vi "Initialize Shared Memory.vi"   [LabVIEW 2013]
doc: "This template VI demonstrates a default initialization that creates and configures a shared memory file in Linux RT. In an unmodified install of Linux RT, the shared memory files will be located at /dev/shm using the name provided to the Initialize Shared Memory VI.\n\nThe template sets the size of the shared memory file to be the size of one page in memory. This avoids page framentation, which may improve performance by reducing the number of interactions with the OS's paging table. However, the size can be set to any value >= 0 if large data sets are required."
uses:
  Classes/Shared Memory/Public/Controls/file mode.ctl
  Classes/Shared Memory/Shared Memory.lvclass
types:
  T1 = typedef "Linux RT IPC.lvlib/Shared Memory.lvlib/Shared Memory.lvclass/file mode.ctl" = enum16{"open", "create/replace"}
  T2 = typedef "Linux RT IPC.lvlib/Shared Memory.lvlib/Shared Memory.lvclass/reference.ctl" = refnum<data-value>
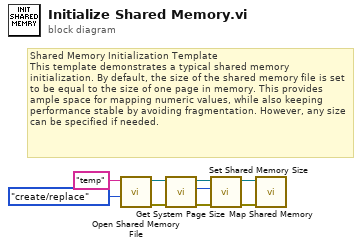
[diagram p0: block diagram]
diagram:
  # "Shared Memory Initialization Template\nThis template demonstrates a typical shared memory initialization. By default, the size of the shared memory file is set to be equal to the size of one page in memory. This provides ample space for mapping numeric values, while also keeping performance stable by avoiding fragmentation. However, any size can be specified if needed."
  n1 = call "Open Shared Memory File.vi"("file mode (open)"=file_mode."create/replace" ("file mode (default: open)"), "shared memory name"="temp") -> ("error out"=w6:errorcluster, "shared memory out"=w7:T2)  [unwired: 8 in]
  n2 = call "Get System Page Size.vi"("error in (no error)"=w6, "shared memory in"=w7) -> ("error out"=w1:errorcluster, "page size (bytes)"=w2:u32, "shared memory out"=w5:T2)  [unwired: 7 in]
  n3 = call "Set Shared Memory Size.vi"("error in (no error)"=w1, "size (bytes)"=w2, "shared memory in"=w5) -> ("error out"=w3:errorcluster, "shared memory out"=w4:T2)  [unwired: 7 in]
  n4 = call "Map Shared Memory.vi"("error in (no error)"=w3, "shared memory in"=w4) -> ()  [unwired: 7 in, 3 out]
